vi "FID Rohwerte kalibrieren.vi"(6 "CAL-Daten":T1={"CH4 Null"=0.0, "CH4 Steil"=[1.0, 1.0, 1.0, 1.0], "THC Null"=0.0, "THC Steil"=[1.0, 1.0, 1.0, 1.0], "NMHC Null"=0.0, "NMHC Steil"=[1.0, 1.0, 1.0, 1.0]}, 8 "Aktuelle MB":i32, 11 "GasValue":sgl[](array[numeric])) -> (3 "Kalibrierte Rohwerte":sgl[](array[numeric]))   [LabVIEW 2020, in "ABB-EL3000.lvlib" / "FID.lvlib" / "FID Kalibrierung.lvlib"]
uses:
  FID Kalibrierung.lvlib
  Allgemeine VI/CAL-Daten FID.ctl
  Allgemeine VI/Allgemeine VI.lvlib
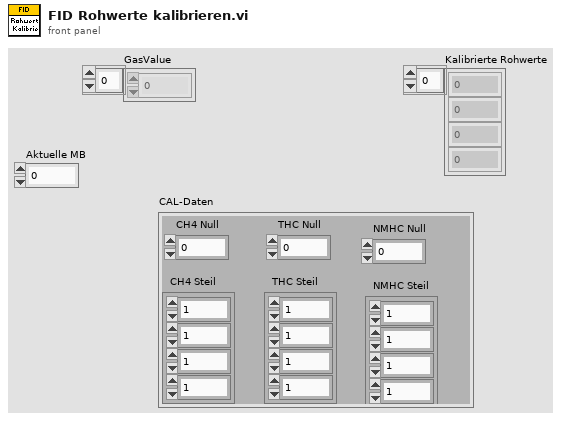
[diagram p1: front panel]
types:
  T1 = typedef "ABB-EL3000.lvlib/Allgemeine VI.lvlib/CAL-Daten FID.ctl" = cluster{"CH4 Null":sgl, "CH4 Steil":sgl[], "THC Null":sgl, "THC Steil":sgl[], "NMHC Null":sgl, "NMHC Steil":sgl[]}
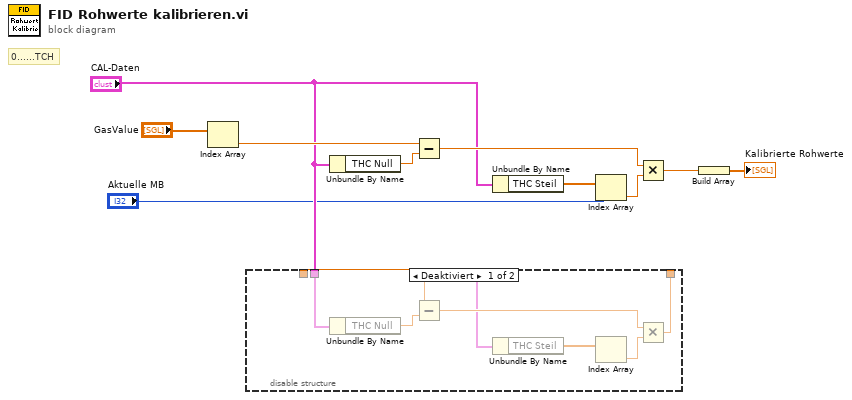
[diagram p0: block diagram]
diagram:
  # "0......TCH"
  n1 = Index Array(array="GasValue") -> (element=w4:sgl)  [unwired: 1 in]
  n2 = disable-structure shown="Deaktiviert" {
    disable-tunnel: _ -> [w13 _]
    disable-tunnel: "CAL-Daten" -> [w12 _]
    disable-tunnel: [w11 _] -> _
    frame Disabled {
      n3 = Unbundle By Name(w12) -> ("THC Null"=w14:sgl)
      n4 = Subtract(x=w13, y=w14) -> (x-y=w15:sgl)
      n5 = Unbundle By Name(w12) -> ("THC Steil"=w16:sgl[])
      n6 = Index Array(array=w16) -> (element=w17:sgl)  [unwired: 1 in]
      n7 = Multiply(x=w15, y=w17) -> (x*y=w11:sgl)
    }
    frame Enabled {
    }
  }
  n8 = Unbundle By Name("CAL-Daten") -> ("THC Null"=w7:sgl)
  n9 = Subtract(x=w4, y=w7) -> (x-y=w8:sgl)
  n10 = Unbundle By Name("CAL-Daten") -> ("THC Steil"=w9:sgl[])
  n11 = Index Array(array=w9, index="Aktuelle MB") -> (element=w10:sgl)
  n12 = Multiply(x=w8, y=w10) -> (x*y=w2:sgl)
  n13 = Build Array(w2) -> (→"Kalibrierte Rohwerte":sgl[])
